vi "Set Transfers.vi"(10 "Transfers":refnum<class "DSF.Engine.Transfer.lvclass">[](array[class]), 11 "Cache in":refnum<class "Memory Cache.lvclass">) -> (3 "Cache out":refnum<class "Memory Cache.lvclass">)   [LabVIEW 2017, in "Data Sharing Framework Engine.lvlib" / "Memory Cache.lvclass"]
uses:
  Memory Cache.lvclass
  old/dsf core/Source/Engine/Classes/Transfer/DSF.Engine.Transfer.lvclass
  Memory Cache.lvclass/Memory Cache.ctl
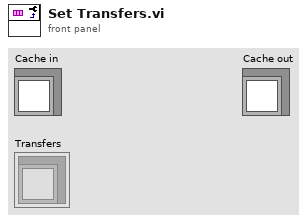
[diagram p1: front panel]
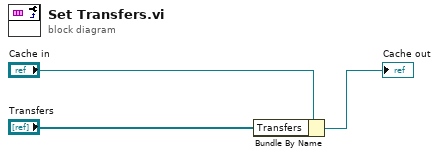
[diagram p0: block diagram]
diagram:
  n1 = Bundle By Name(cluster="Cache in", "Transfers"="Transfers") -> (→"Cache out":refnum<class "Memory Cache.lvclass">)
